vi "Node Info Service Async.vi"(11 "InfoService in":refnum<class "InfoService.lvclass">) -> ()   [LabVIEW 2020, in "Vecto.lvlib" / "InfoService.lvclass"]
uses:
  InfoService.lvclass
  Data.ctl
  Node Info.ctl
  Task Info.ctl
  InfoService.lvclass/InfoService.ctl
  NodeInfoValue/NodeInfoValue.lvclass/NodeInfoValue.ctl
  NodeInfoValue/NodeInfoValue.lvclass
  C:/Program Files (x86)/National Instruments/LabVIEW 2020/vi.lib/IlluminatedG/IG Promises/Promises/Value/Value.lvclass
  Vecto.lvlib
  <vilib>/IlluminatedG/IG Promises/Promises/Promise/Promise.lvclass
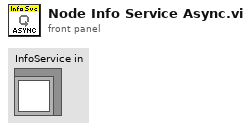
[diagram p1: front panel]
types:
  T1 = typedef "Vecto.lvlib/InfoService.lvclass/Data.ctl" = cluster{"Node Info":T2, "Task Status":map{string, string}}
  T2 = typedef "Vecto.lvlib/Node Info.ctl" = cluster{"Name":string, "ID":i32, "Status":string, "SWVersion":string, "ConfigVersion":string, "Tasks":T3[]}
  T3 = typedef "Vecto.lvlib/Task Info.ctl" = cluster{"Name":string, "Status":string}
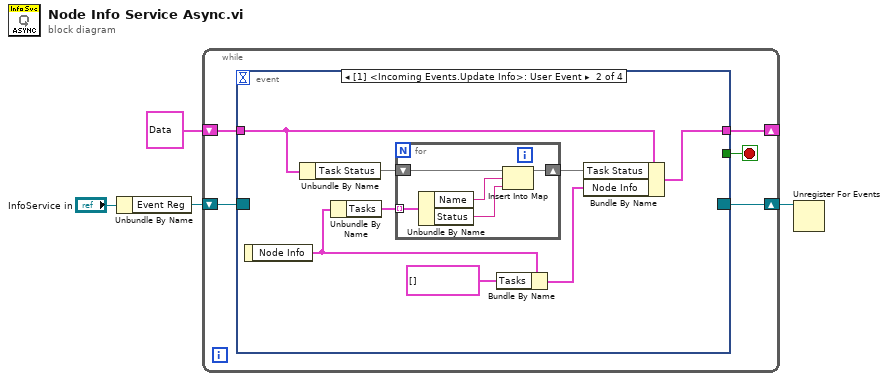
[diagram p0: block diagram]
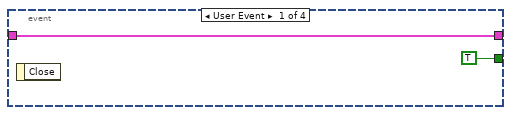
[diagram p2: hidden frame]
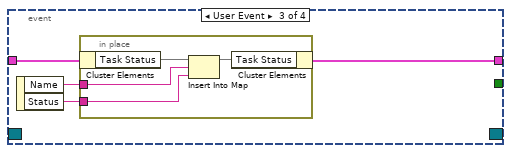
[diagram p3: hidden frame]
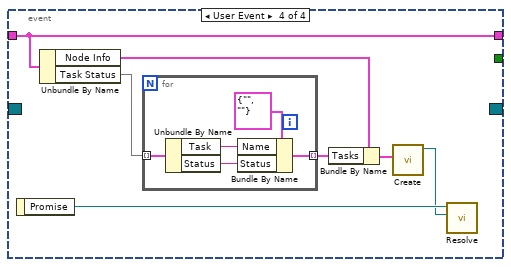
[diagram p4: hidden frame]
diagram:
  n1 = Unbundle By Name("InfoService in") -> ("Event Reg"=w3:refnum<event-registration>)
  n2 = while {
    shift-right: [w8] -> w2
    shift-left: w3 -> [w9]
    shift-right: [w5] -> _
    shift-left: T1 {"Node Info"={"Name"="", "ID"=0, "Status"="", "SWVersion"="", "ConfigVersion"="", "Tasks"=[]}, "Task Status"={}} ("Data") -> [w6]
    stop <- w7 stop-if-true
    n3 = event shown="[1] <Incoming Events.Update Info>: User Event" {
      selector: w9 -> [_ _ _ _]
      dyn-events: [_ _ _ _] -> w8
      timeout: _ -> [_ _ _ _]
      tunnel: [TRUE _ _ _] -> w7
      tunnel: w6 -> [w10 w15 w28 w39]
      tunnel: [w10 w12 w25 w39] -> w5
      event User Event {
        n4 = event-data() -> ()  [unwired: 1 in, 1 out]
      }
      event User Event {
        n5 = event-data() -> ("Node Info"=w19:T2)  [unwired: 1 in]
        n6 = Unbundle By Name(w15) -> ("Task Status"=w17:map{string, string})
        n7 = Unbundle By Name(w19) -> ("Tasks"=w16:T3[])
        n8 = for {
          shift-right: [w20] -> w14
          shift-left: w17 -> [w23]
          tunnel: w16 -> [w24] mode=indexing
          n9 = Unbundle By Name(w24) -> ("Name"=w22:string, "Status"=w21:string)
          n10 = Insert Into Map(map in=w23, key=w22, value=w21) -> (map out=w20:map{string, string})  [unwired: 2 out]
        }
        n11 = Bundle By Name(cluster=w19, "Tasks"=T3[] []) -> (w13:T2)
        n12 = Bundle By Name(cluster=w15, "Task Status"=w14, "Node Info"=w13) -> (w12:T1)
      }
      event User Event {
        n13 = event-data() -> ("Name"=w27:string, "Status"=w26:string)  [unwired: 1 in]
        n14 = in-place {
          in-place-border: w27 -> [w31]
          in-place-border: w26 -> [w30]
          n15 = in-place-cluster #1(w28) -> ("Task Status"=w32:map{string, string})
          n16 = Insert Into Map(map in=w32, key=w31, value=w30) -> (map out=w29:map{string, string})  [unwired: 2 out]
          n17 = in-place-cluster #1("Task Status"=w29) -> (w25:T1)
        }
      }
      event User Event {
        n18 = event-data() -> ("Promise"=w34:refnum<class "Promise.lvclass">)  [unwired: 1 in]
        n19 = Unbundle By Name(w39) -> ("Node Info"=w37:T2, "Task Status"=w38:map{string, string})
        n20 = for {
          tunnel: w38 -> [w44] mode=indexing
          tunnel: [w40] -> w36 mode=indexing
          n21 = Unbundle By Name(w44) -> ("Task"=w42:string, "Status"=w41:string)
          n22 = Bundle By Name(cluster=T3 {"Name"="", "Status"=""} ("Task Info"), "Name"=w42, "Status"=w41) -> (w40:T3)
        }
        n23 = Bundle By Name(cluster=w37, "Tasks"=w36) -> (w35:T2)
        n24 = call "Create.vi"("Node Info"=w35) -> ("NodeInfoValue out"=w33:refnum<class "NodeInfoValue.lvclass">)  [unwired: 10 in]
        n25 = call <vilib>:"Resolve.vi"("Result"=w33, "Promise in"=w34) -> ()  [unwired: 8 in, 2 out]
      }
    }
  }
  n26 = Unregister For Events(event registration refnum=w2) -> ()  [unwired: 1 in, 1 out]
